vi "创建队列.vi"() -> (0 "错误输出":errorcluster, 2 "结束位队列":refnum<queue>, 3 "数据队列":refnum<queue>)   [LabVIEW 2020]
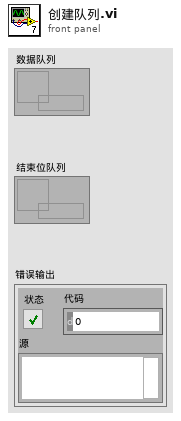
[diagram p1: front panel]
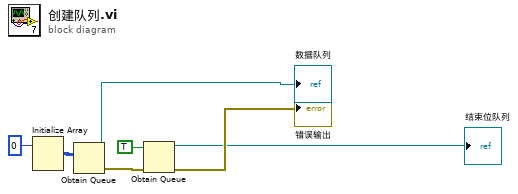
[diagram p0: block diagram]
diagram:
  n1 = Initialize Array(0) -> (w3:i32[][])  [unwired: 2 in]
  n2 = Obtain Queue(element data type=w3) -> (queue out=→"数据队列":refnum<queue>, error out=w4:errorcluster)  [unwired: 4 in, 1 out]
  n3 = Obtain Queue(element data type=TRUE, error in (no error)=w4) -> (queue out=→"结束位队列":refnum<queue>, error out=→"错误输出":errorcluster)  [unwired: 3 in, 1 out]
